vi "Go to Init.vi"(8 "error in (no error)":errorcluster, 11 "Test State in":refnum<class "Test State.lvclass">) -> (0 "error out":errorcluster, 3 "State Actor.lvclass":refnum<class "State Actor.lvclass">)   [LabVIEW 2024, in "Test States.lvlib" / "Test State.lvclass"]
uses:
  Test State.lvclass
  C:/Program Files/National Instruments/LabVIEW 2024/vi.lib/ni/Actors/State Actor/State Actor/State Actor.lvclass
  <vilib>/ni/Actors/State Actor/State Actor/State Actor.lvclass
  Init/Init.lvclass
  G:/Leveling/LabVIEW/Learning/Actor Framework/actor-state-machine/Test States/Test State/Test State.lvclass
  Test State.lvclass/Test State.ctl
  C:/Program Files/National Instruments/LabVIEW 2024/vi.lib/ActorFramework/Actor/Actor.lvclass
  G:/Leveling/LabVIEW/Learning/Actor Framework/actor-state-machine/Test States/Init/Init.lvclass
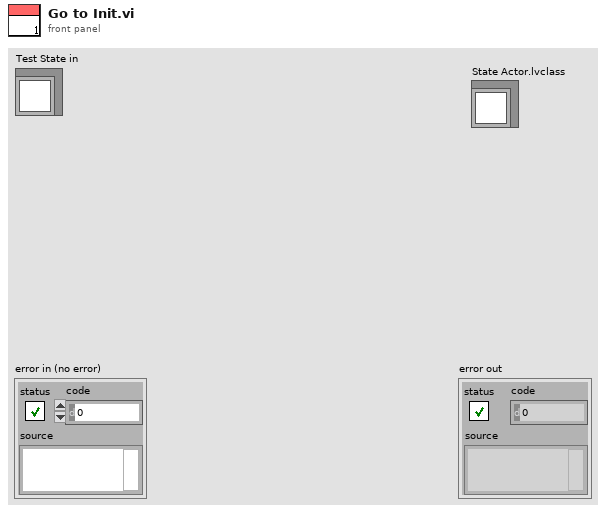
[diagram p1: front panel]
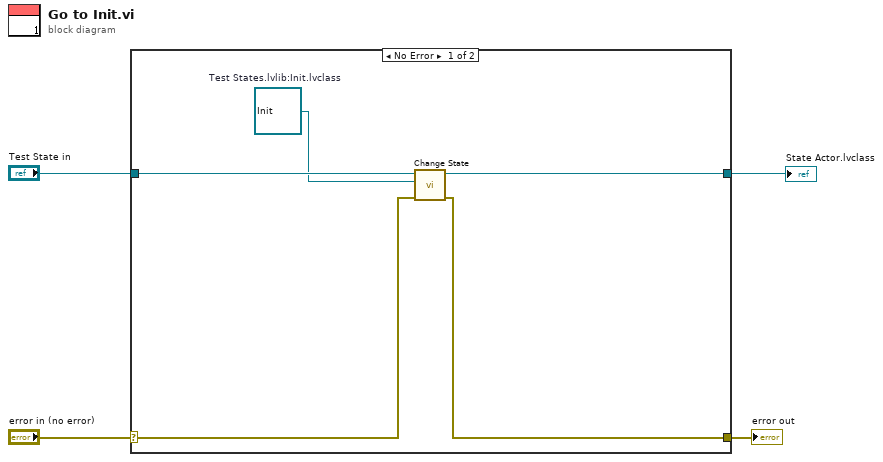
[diagram p0: block diagram]
diagram:
  n1 = case shown="No Error" "error in (no error)" {
    selector: "error in (no error)" -> [w9 w11]
    tunnel: [w6 w11] -> w3
    tunnel: [w5 w10] -> w1
    tunnel: "Test State in" -> [w8 w10]
    frame No Error {
      w7 = refnum<class "Init.lvclass"> refnum  # Test States.lvlib:Init.lvclass
      n2 = call <vilib>:"Change State.vi"("error in (no error)"=w9, "New State in"=w7, "State in"=w8) -> ("error out"=w6:errorcluster, "State out"=w5:refnum<class "State Actor.lvclass">)  [unwired: 7 in]
    }
    frame Error {
    }
  }
  "error out" <- w3
  "State Actor.lvclass" <- w1
